vi "Add SubSymbols to Symbol Map.vi"(8 "error in (no error)":errorcluster, 9 ".NET TcAdsSymbolInfo":refnum<k24>, 11 "Symbol Map in":variant) -> (0 "error out":errorcluster, 3 "Symbol Map out":variant)   [LabVIEW 2018, in "TwinCAT ADS.lvclass"]
uses:
  TwinCAT ADS.lvclass
  TwinCAT.Ads
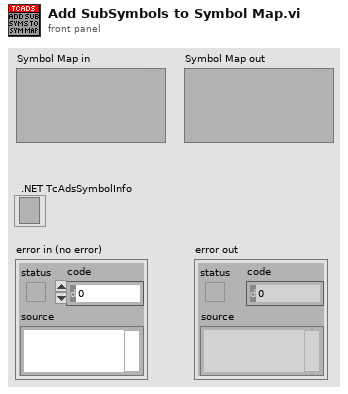
[diagram p1: front panel]
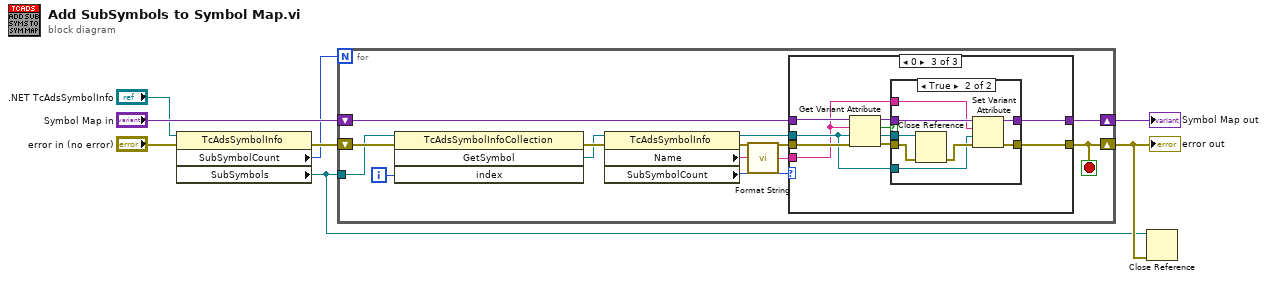
[diagram p0: block diagram]
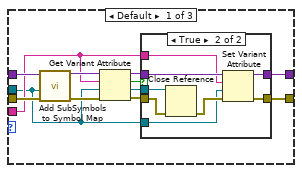
[diagram p2: hidden frame]
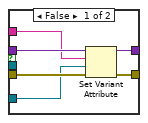
[diagram p3: hidden frame]
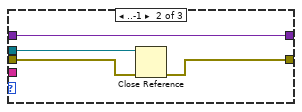
[diagram p4: hidden frame]
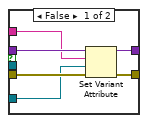
[diagram p5: hidden frame]
diagram:
  n1 = property class="TcAdsSymbolInfo"(reference=".NET TcAdsSymbolInfo", error in="error in (no error)") -> (error out=w4:errorcluster, "SubSymbolCount"=w3:i32, "SubSymbols"=w1:refnum<k24>)  [unwired: 1 out]
  n2 = for {
    N: w3 -> [_]
    shift-right: [w13] -> w6
    shift-left: "Symbol Map in" -> [w19]
    shift-right: [w9] -> w2
    shift-left: w4 -> [w21]
    tunnel: w1 -> [w12]
    i -> [w20]
    stop <- w9 stop-if-true
    n3 = invoke class="TcAdsSymbolInfoCollection" method="GetSymbol"(reference=w12, error in=w21, "index"=w20) -> (error out=w18:errorcluster, "GetSymbol"=w17:refnum<k24>)  [unwired: 1 in, 2 out]
    n4 = property class="TcAdsSymbolInfo"(reference=w17, error in=w18) -> (reference out=w14:refnum<k24>, error out=w16:errorcluster, "Name"=w11:string, "SubSymbolCount"=w15:i32)
    n5 = call "Format String.vi"("String"=w11) -> ("Formated String"=w10:string)
    n6 = case shown="0" w15 {
      tunnel: w19 -> [w33 w51 w58]
      tunnel: w16 -> [w32 w50 w59]
      tunnel: w14 -> [w24 w49 w53]
      tunnel: w10 -> [w25 _ w52]
      tunnel: [w23 w48 w60] -> w9
      tunnel: [w22 w51 w61] -> w13
      frame Default {
        n7 = call "Add SubSymbols to Symbol Map.vi"("error in (no error)"=w32, ".NET TcAdsSymbolInfo"=w24, "Symbol Map in"=w33) -> ("error out"=w26:errorcluster, "Symbol Map out"=w27:variant)  [unwired: 7 in]
        n8 = Get Variant Attribute(Variant=w27, name=w25, default value (empty Variant)=w24, error in=w26) -> (duplicate Variant=w30:variant, found=w29:bool, value=w28:refnum<k24>, error out=w31:errorcluster)
        n9 = case shown="True" w29 {
          tunnel: w30 -> [w39 w45]
          tunnel: w31 -> [w37 w46]
          tunnel: [w38 w42] -> w22
          tunnel: [w36 w43] -> w23
          tunnel: w28 -> [_ w47]
          tunnel: w24 -> [w35 w41]
          tunnel: w25 -> [w34 w40]
          frame False {
            n10 = Set Variant Attribute(Variant=w39, name=w34, value=w35, error in=w37) -> (Variant out=w38:variant, error out=w36:errorcluster)  [unwired: 1 out]
          }
          frame True {
            n11 = Close Reference(reference=w47, error in (no error)=w46) -> (error out=w44:errorcluster)
            n12 = Set Variant Attribute(Variant=w45, name=w40, value=w41, error in=w44) -> (Variant out=w42:variant, error out=w43:errorcluster)  [unwired: 1 out]
          }
        }
      }
      frame ..-1 {
        n13 = Close Reference(reference=w49, error in (no error)=w50) -> (error out=w48:errorcluster)
      }
      frame 0 {
        n14 = Get Variant Attribute(Variant=w58, name=w52, default value (empty Variant)=w53, error in=w59) -> (duplicate Variant=w56:variant, found=w55:bool, value=w54:refnum<k24>, error out=w57:errorcluster)
        n15 = case shown="True" w55 {
          tunnel: w56 -> [w67 w73]
          tunnel: w57 -> [w65 w74]
          tunnel: [w66 w70] -> w61
          tunnel: [w64 w71] -> w60
          tunnel: w54 -> [_ w75]
          tunnel: w53 -> [w63 w69]
          tunnel: w52 -> [w62 w68]
          frame False {
            n16 = Set Variant Attribute(Variant=w67, name=w62, value=w63, error in=w65) -> (Variant out=w66:variant, error out=w64:errorcluster)  [unwired: 1 out]
          }
          frame True {
            n17 = Close Reference(reference=w75, error in (no error)=w74) -> (error out=w72:errorcluster)
            n18 = Set Variant Attribute(Variant=w73, name=w68, value=w69, error in=w72) -> (Variant out=w70:variant, error out=w71:errorcluster)  [unwired: 1 out]
          }
        }
      }
    }
  }
  "error out" <- w2
  "Symbol Map out" <- w6
  n19 = Close Reference(reference=w1, error in (no error)=w2) -> ()  [unwired: 1 out]
